vi "Generate CSV Report combined.vi"(8 "error in":errorcluster, 9 "Variant":string, 10 "Results":T1[](array[typedef]), 11 "Program Data":T2) -> (0 "error out":errorcluster)   [LabVIEW 2025]
uses:
  <vilib>/Utility/file.llb/Write Delimited Spreadsheet (string).vi
  Controls/ProgramData.ctl
  Controls/ResultData.ctl
  Controls/TestTypes.ctl
  Communication Handle/API/Commands.ctl
  Controls/References.ctl
  Controls/paths.ctl
  Controls/Section4 variables.ctl
  Controls/Variants.ctl
  Controls/Test Data.ctl
  Communication Handle/Controls/CAN Payload.ctl
  Communication Handle/API/Notifier Data.ctl
  Communication Handle/Controls/CAN Sending Data.ctl
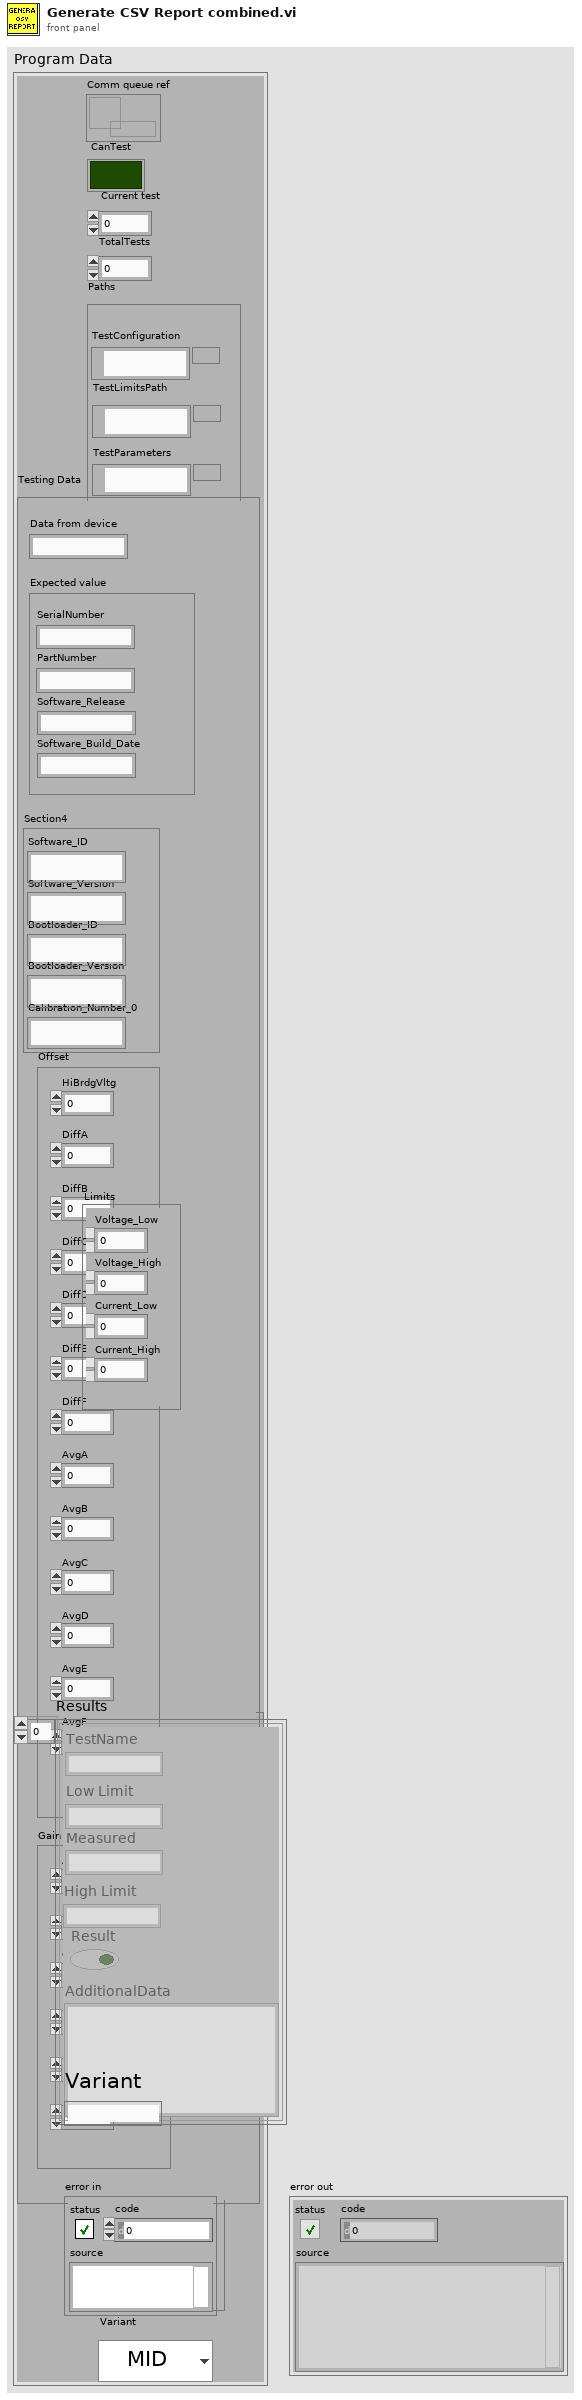
[diagram p1: front panel]
types:
  T1 = typedef "ResultData.ctl" = cluster{"TestName":string, "Measured":string, "Result":bool, "Low Limit":string, "High Limit":string, "AdditionalData":string}
  T2 = typedef "ProgramData.ctl" = cluster{"Current test":i32, "TotalTests":i32, "TestNames":string[], "CurrentTest":string, "TestStatus":bool, "C Serial Number":string, "Reader":refnum<visa-resource-name>, "CanTest":bool, "TestTypes":T3[], "Commands":T4[], "AdditionalData":bool[], "Log result":bool[], "References":T5, "Paths":T6, "Section4":T7, "Variant":T8, "Testing Data":T9, "Comm queue ref":refnum<queue>, "Limits":cluster{"Voltage_Low":dbl, "Voltage_High":dbl, "Current_Low":dbl, "Current_High":dbl}}
  T3 = typedef "TestTypes.ctl" = enum16{"CHCK", "WAIT", "PERI", "TEST", "COMM", "CONN", "CPWR", "DPWR"}
  T4 = typedef "Commands.ctl" = enum16{"Nexteer connect", "Write Polarity", "Write BEMF", "Write Torque Scale Sensors T1", "Write Torque Scale Sensors T2", "Trim HW Torque Sensors T1", "Trim HW Torque Sensors T2", "Read HW Torque Trim Performed Sensors T1", "Read HW Torque Trim Performed Sensors T2", "Write EOL Offset values to defaults", "Write EOL Gain values to defaults", "Write Serial Number", "Write Hardware Part Number", "Write EPS Serial Number", "Read MEC Counter", "MCU Reset", "Read System State", "Read First Motor Position", "Manufacturing Diagnostic Defeat", "Perform Current Offset ", "Current Offset Status", "Enable Engine Run", "Perform Current Gain ", "Current Gain Status", "Disable Torque Ramp Down ", "Disable Engine Run", "Set Vehicle Speed Override", "Read Offset Values Using FD F5", "Read Gain Values Using FD F4", "Clear Nexteer NTCs", "Read Second Motor Position", "Read ECU Software ID", "Read Internal Software Version", "Read Bootloader ID", "Read Bootloader Software Version", "Read Calibration Release 0", "Read Calibration Release 1", "Read Calibration Release 2", "Read Temperature  ", "Battery Voltage  ", "Read Motor Angle 0", "Read Motor Angle 1 ", "Set Motor Torque Command ", "Read Motor Current   ", "Stop Motor Torque Command", "Read NTCs", "Read Serial Number", "Read HW Part Number", "Read Polarity", "Set NVM Access Defeat", "Read Software Release", "Read Software Build Date", "Write Single Inverter Hardware value", "Write Dual Inverter Hardware value", "Read Single Inverter HW Value", "Read Dual Inverter HW Value", "Write MEC Counter FE", "Write MEC Counter FF", "Read BEMF", "Read Torque 1 FDB6", "Read Torque 2 FDB7", "Read Torque Trim 1 FDB4", "Read Torque Trim 2 FDB5", "Write Torque Trim 1 FDB4", "Write Torque Trim 2 FDB5", "XCP connect", "Read HW Torque T1", "Read HW Torque T2", "Read Motor Speed "}
  T5 = typedef "References.ctl" = cluster{"Scanner":refnum<visa-resource-name>, "NI_CAN":refnum<visa-resource-name>, "Arduino_Nano":refnum<visa-resource-name>, "DUT PS":refnum<visa-resource-name>, "CalPS1":refnum<visa-resource-name>, "CalPS2":refnum<visa-resource-name>}
  T6 = typedef "paths.ctl" = cluster{"TestConfiguration":path, "TestLimitsPath":path, "TestParameters":path, "CSVconf":path}
  T7 = typedef "Section4 variables.ctl" = cluster{"Software_ID":string, "Software_Version":string, "Bootloader_ID":string, "Bootloader_Version":string, "Calibration_Number_0":string}
  T8 = typedef "Variants.ctl" = enum16{"MID", "HI_RHD", "HI_LHD"}
  T9 = typedef "Test Data.ctl" = cluster{"Section4":T7, "Expected value":cluster{"SerialNumber":string, "PartNumber":string, "Software_Release":string, "Software_Build_Date":string}, "Data from device":string, "Offset":cluster{"HiBrdgVltg":dbl, "DiffA":dbl, "DiffB":dbl, "DiffC":dbl, "DiffD":dbl, "DiffE":dbl, "DiffF":dbl, "AvgA":dbl, "AvgB":dbl, "AvgC":dbl, "AvgD":dbl, "AvgE":dbl, "AvgF":dbl}, "Gain":cluster{"A":dbl, "B":dbl, "C":dbl, "D":dbl, "E":dbl, "F":dbl}}
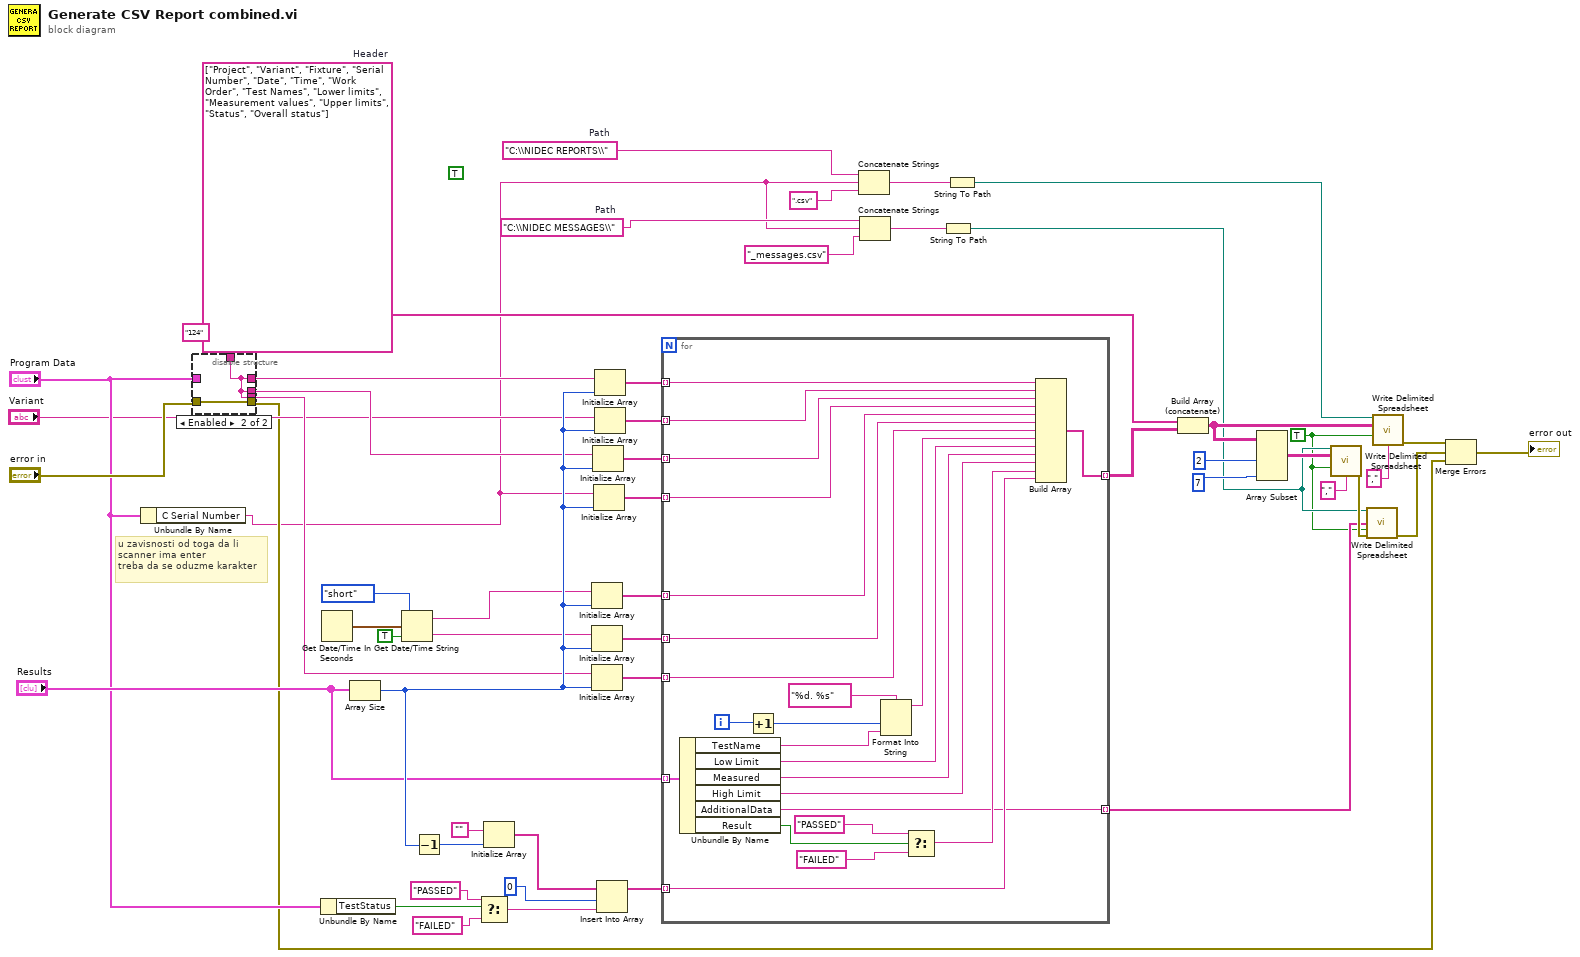
[diagram p0: block diagram]
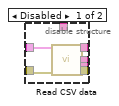
[diagram p2: hidden frame]
diagram:
  w2 = "C:\\NIDEC MESSAGES\\"  # Path
  (unwired) TRUE ("replace all? (F)")
  w3 = TRUE ("append to file? (new file:F)")
  w17 = "C:\\NIDEC REPORTS\\"  # Path
  w46 = string[] ["Project", "Variant", "Fixture", "Serial Number", "Date", "Time", "Work Order", "Test Names", "Lower limits", "Measurement values", "Upper limits", "Status", "Overall status"]  # Header
  # "u zavisnosti od toga da li\nscanner ima enter\ntreba da se oduzme karakter"
  n1 = Unbundle By Name("Program Data") -> ("C Serial Number"=w1:string)
  n2 = disable-structure shown="Enabled" {
    disable-tunnel: [w60 w61] -> w36
    disable-tunnel: [w59 w61] -> w35
    disable-tunnel: [w58 w61] -> w34
    disable-tunnel: "error in" -> [w57 w62]
    disable-tunnel: "Program Data" -> [w56 _]
    disable-tunnel: [w55 w62] -> w14
    disable-tunnel: "124" ("Project") -> [_ w61]
    frame Disabled {
      n3 = call "Read CSV data.vi"("Program Data"=w56, "error in"=w57) -> ("Project"=w60:string, "Fixture"=w59:string, "Work_Order"=w58:string, "error out"=w55:errorcluster)  [unwired: 9 in, 1 out]
    }
    frame Enabled {
    }
  }
  n4 = Unbundle By Name("Program Data") -> ("TestStatus"=w29:bool)
  n5 = Get Date/Time In Seconds() -> (seconds since 1Jan1904=w22:timestamp)
  n6 = Array Size(array="Results") -> (size(s)=w39:i32)
  n7 = Get Date/Time String(date format (0)=enum16{"short", "long", "abbreviated"}."short", seconds (now)=w22, want seconds? (F)=TRUE) -> (date string=w21:string, time string=w20:string)
  n8 = Decrement(x=w39) -> (x-1=w43:i32)
  n9 = Select(t="PASSED" ("LimitHigh"), s=w29, f="FAILED" ("LimitHigh")) -> (s? t:f=w28:string)
  n10 = Initialize Array("", w43) -> (w38:string[])
  n11 = Initialize Array(w21, w39) -> (w51:string[])
  n12 = Initialize Array(w20, w39) -> (w50:string[])
  n13 = Initialize Array(w34, w39) -> (w41:string[])
  n14 = Initialize Array(w35, w39) -> (w52:string[])
  n15 = Initialize Array(w1, w39) -> (w47:string[])
  n16 = Initialize Array(w36, w39) -> (w54:string[])
  n17 = Initialize Array("Variant", w39) -> (w53:string[])
  n18 = Insert Into Array(array=w38, index=0, new element=w28) -> (w49:string[])
  n19 = for {
    tunnel: w54 -> [w84] mode=indexing
    tunnel: w53 -> [w83] mode=indexing
    tunnel: w52 -> [w82] mode=indexing
    tunnel: w47 -> [w81] mode=indexing
    tunnel: w51 -> [w80] mode=indexing
    tunnel: w50 -> [w79] mode=indexing
    tunnel: w49 -> [w64] mode=indexing
    tunnel: [w85] -> w45 mode=indexing
    tunnel: w41 -> [w78] mode=indexing
    tunnel: "Results" -> [w77] mode=indexing
    tunnel: [w63] -> w4 mode=indexing
    i -> [w66]
    n20 = Unbundle By Name(w77) -> ("TestName"=w68:string, "Low Limit"=w76:string, "Measured"=w75:string, "High Limit"=w74:string, "AdditionalData"=w63:string, "Result"=w71:bool)
    n21 = Increment(x=w66) -> (x+1=w69:i32)
    n22 = Format Into String(format string="%d. %s", w69, w68) -> (resulting string=w67:string)  [unwired: 2 in, 1 out]
    n23 = Select(t="PASSED" ("LimitHigh"), s=w71, f="FAILED" ("LimitHigh")) -> (s? t:f=w65:string)
    n24 = Build Array(w84, w83, w82, w81, w80, w79, w78, w67, w76, w75, w74, w65, w64) -> (w85:string[])
  }
  n25 = Concatenate Strings(w17, w1, ".csv" ("string")) -> (w18:string)
  n26 = Concatenate Strings(w2, w1, "_messages.csv" ("string")) -> (w15:string)
  n27 = String To Path(string=w15) -> (path=w5:path)
  n28 = String To Path(string=w18) -> (path=w44:path)
  n29 = Build Array (concatenate)(w46, w45) -> (w13:string[][])
  n30 = Array Subset(array=w13, length (row)=2 ("length"), length (col)=7 ("length")) -> (w8:string[][])  [unwired: 2 in]
  n31 = call-poly <vilib>:"Write Delimited Spreadsheet.vi"("file path (dialog if empty)"=w5, "2D data"=w8, "append to file? (new file:F)"=w3, "delimiter (\\t)"="," ("delimiter (\\t)")) -> ("error out"=w7:errorcluster)  [unwired: 10 in, 1 out]
  n32 = call-poly <vilib>:"Write Delimited Spreadsheet.vi"("file path (dialog if empty)"=w5, "1D data"=w4, "append to file? (new file:F)"=w3, "error in (no error)"=w7) -> ("error out"=w6:errorcluster)  [unwired: 10 in, 1 out]
  n33 = call-poly <vilib>:"Write Delimited Spreadsheet.vi"("file path (dialog if empty)"=w44, "2D data"=w13, "append to file? (new file:F)"=w3, "delimiter (\\t)"="," ("delimiter (\\t)")) -> ("error out"=w33:errorcluster)  [unwired: 10 in, 1 out]
  n34 = Merge Errors(w33, w6, w14) -> (→"error out":errorcluster)
